vi "Graham Scan Point to Graph Point.vi"(1 "Array":T1[](array[typedef])) -> (0 "Array Out":cluster{"X":i32, "Y":i32}[](array[cluster]))   [LabVIEW 2018]
uses:
  Graham Scan Point.ctl
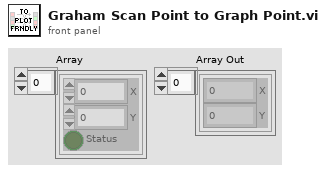
[diagram p1: front panel]
types:
  T1 = typedef "Graham Scan Point.ctl" = cluster{"X":i32, "Y":i32, "Status":bool}
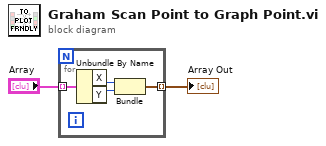
[diagram p0: block diagram]
diagram:
  n1 = for {
    tunnel: "Array" -> [w6] mode=indexing
    tunnel: [w3] -> w1 mode=indexing
    n2 = Unbundle By Name(w6) -> ("X"=w4:i32, "Y"=w5:i32)
    n3 = Bundle("X"=w4, "Y"=w5) -> (w3:cluster{"X":i32, "Y":i32})  [unwired: 1 in]
  }
  "Array Out" <- w1
